vi "String to Number Conversion.vi"() -> ()   [LabVIEW 2020]
panel:
  out "Decimal Number as Double":dbl=3.0 format="%.2f"
  out "Fract/Exp Number":dbl=3.14159265359
  out "Octal Number":u32=3
  out "Hexadecimal Number":i64=3
  out "Decimal Number":i8=3
  in  "Numeric String":string="3.14159265359"
  # "Check the display format for digit length"
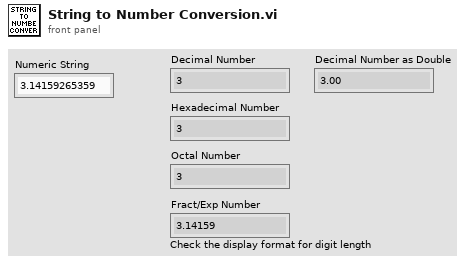
[diagram p1: front panel]
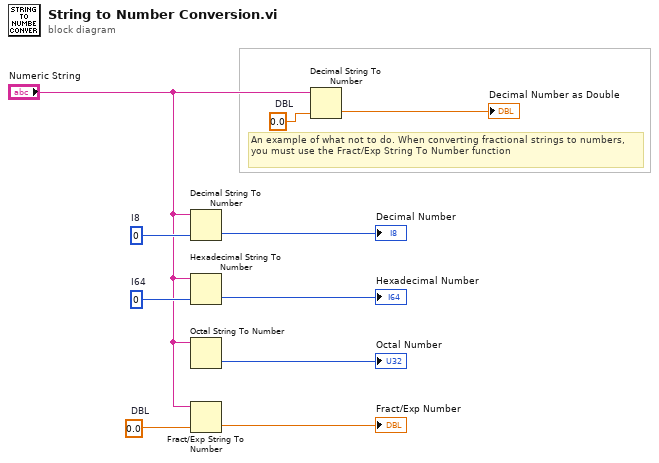
[diagram p0: block diagram]
diagram:
  w3 = 0.0  # DBL
  w9 = i8 0  # I8
  w8 = 0.0  # DBL
  w10 = i64 0  # I64
  # "An example of what not to do. When converting fractional strings to numbers, you must use the Fract/Exp String To Number function"
  n1 = Decimal String To Number(string="Numeric String", default (0L)=w9) -> (number=→"Decimal Number":i8)  [unwired: 1 in, 1 out]
  n2 = Hexadecimal String To Number(string="Numeric String", default (0uL)=w10) -> (number=→"Hexadecimal Number":i64)  [unwired: 1 in, 1 out]
  n3 = Octal String To Number(4:"Numeric String") -> (0:→"Octal Number":u32)  [unwired: 2 in, 1 out]
  n4 = Fract/Exp String To Number(string="Numeric String", default (0 dbl)=w8) -> (number=→"Fract/Exp Number":dbl)  [unwired: 2 in, 1 out]
  n5 = Decimal String To Number(string="Numeric String", default (0L)=w3) -> (number=→"Decimal Number as Double":dbl)  [unwired: 1 in, 1 out]
